vi "Lockin_Amplifier_diag_realtime.vi"(0 "Second":bool, 1 "Sample Number":i32=100000, 2 "all rows":dbl[][](array[numeric]) format="%0.3f", 3 "Cutoff Frequency":dbl=500.0, 4 "dt":dbl=0.0002, 5 "Window (s)":dbl=3.0, 7 "Resolution":dbl=0.0001, 8 "averaging time":dbl=1.0 format="%0.2p", 9 "Error In":errorcluster, 12 "Sampling Freq":dbl=5000.0, 14 "tolerance (Deviation)":dbl=3.0) -> (13 "Error Out":errorcluster, 15 "dLD_RMS":dbl, 16 "LD_RMS":dbl, 17 "Signal Spectrum":cluster{"f0":dbl, "df":dbl, "magnitude":dbl[]}[](graph), 20 "Lock-in R (Vrms)":cluster{dbl[], "Result":dbl[]}(graph), 21 "Lock-in Theta":cluster{dbl[], "Result":dbl[]}(graph), 23 "Time Domain Signal":cluster{"xi used":dbl[], "yi":dbl[]}[](graph), 24 "Phase average":dbl format="%0.2f", 25 "Phase  deviation":dbl format="%0.2f", 27 "Integral":cluster{dbl[], dbl[]}[](graph))   [LabVIEW 2013]
uses:
  <vilib>/gmath/NI_Gmath.lvlib
  <vilib>/Analysis/NI_AALBase.lvlib
panel:
  out "Averaging window":dbl
  in  "Tab Control":T1(tab)
  out "Reference signal / PLL Signal":cluster{"all rows":dbl[], "all rows":dbl[]}[](graph)
  out "Reference Spectrum":cluster{"f0":dbl, "df":dbl, "magnitude":dbl[]}(graph)
  out "Synthetized Spectrum":cluster{"f0":dbl, "df":dbl, "magnitude":dbl[]}(graph)
  in  "t0_ref":dbl
  in  "t0_LD":dbl=0.0001
  out "LD Spectrum":cluster{"f0":dbl, "df":dbl, "magnitude":dbl[]}(graph)
  out "LD Signal":cluster{"all rows":dbl[], "all rows":dbl[]}[](graph)
  out "Tolerance Level":dbl
  out "average":dbl
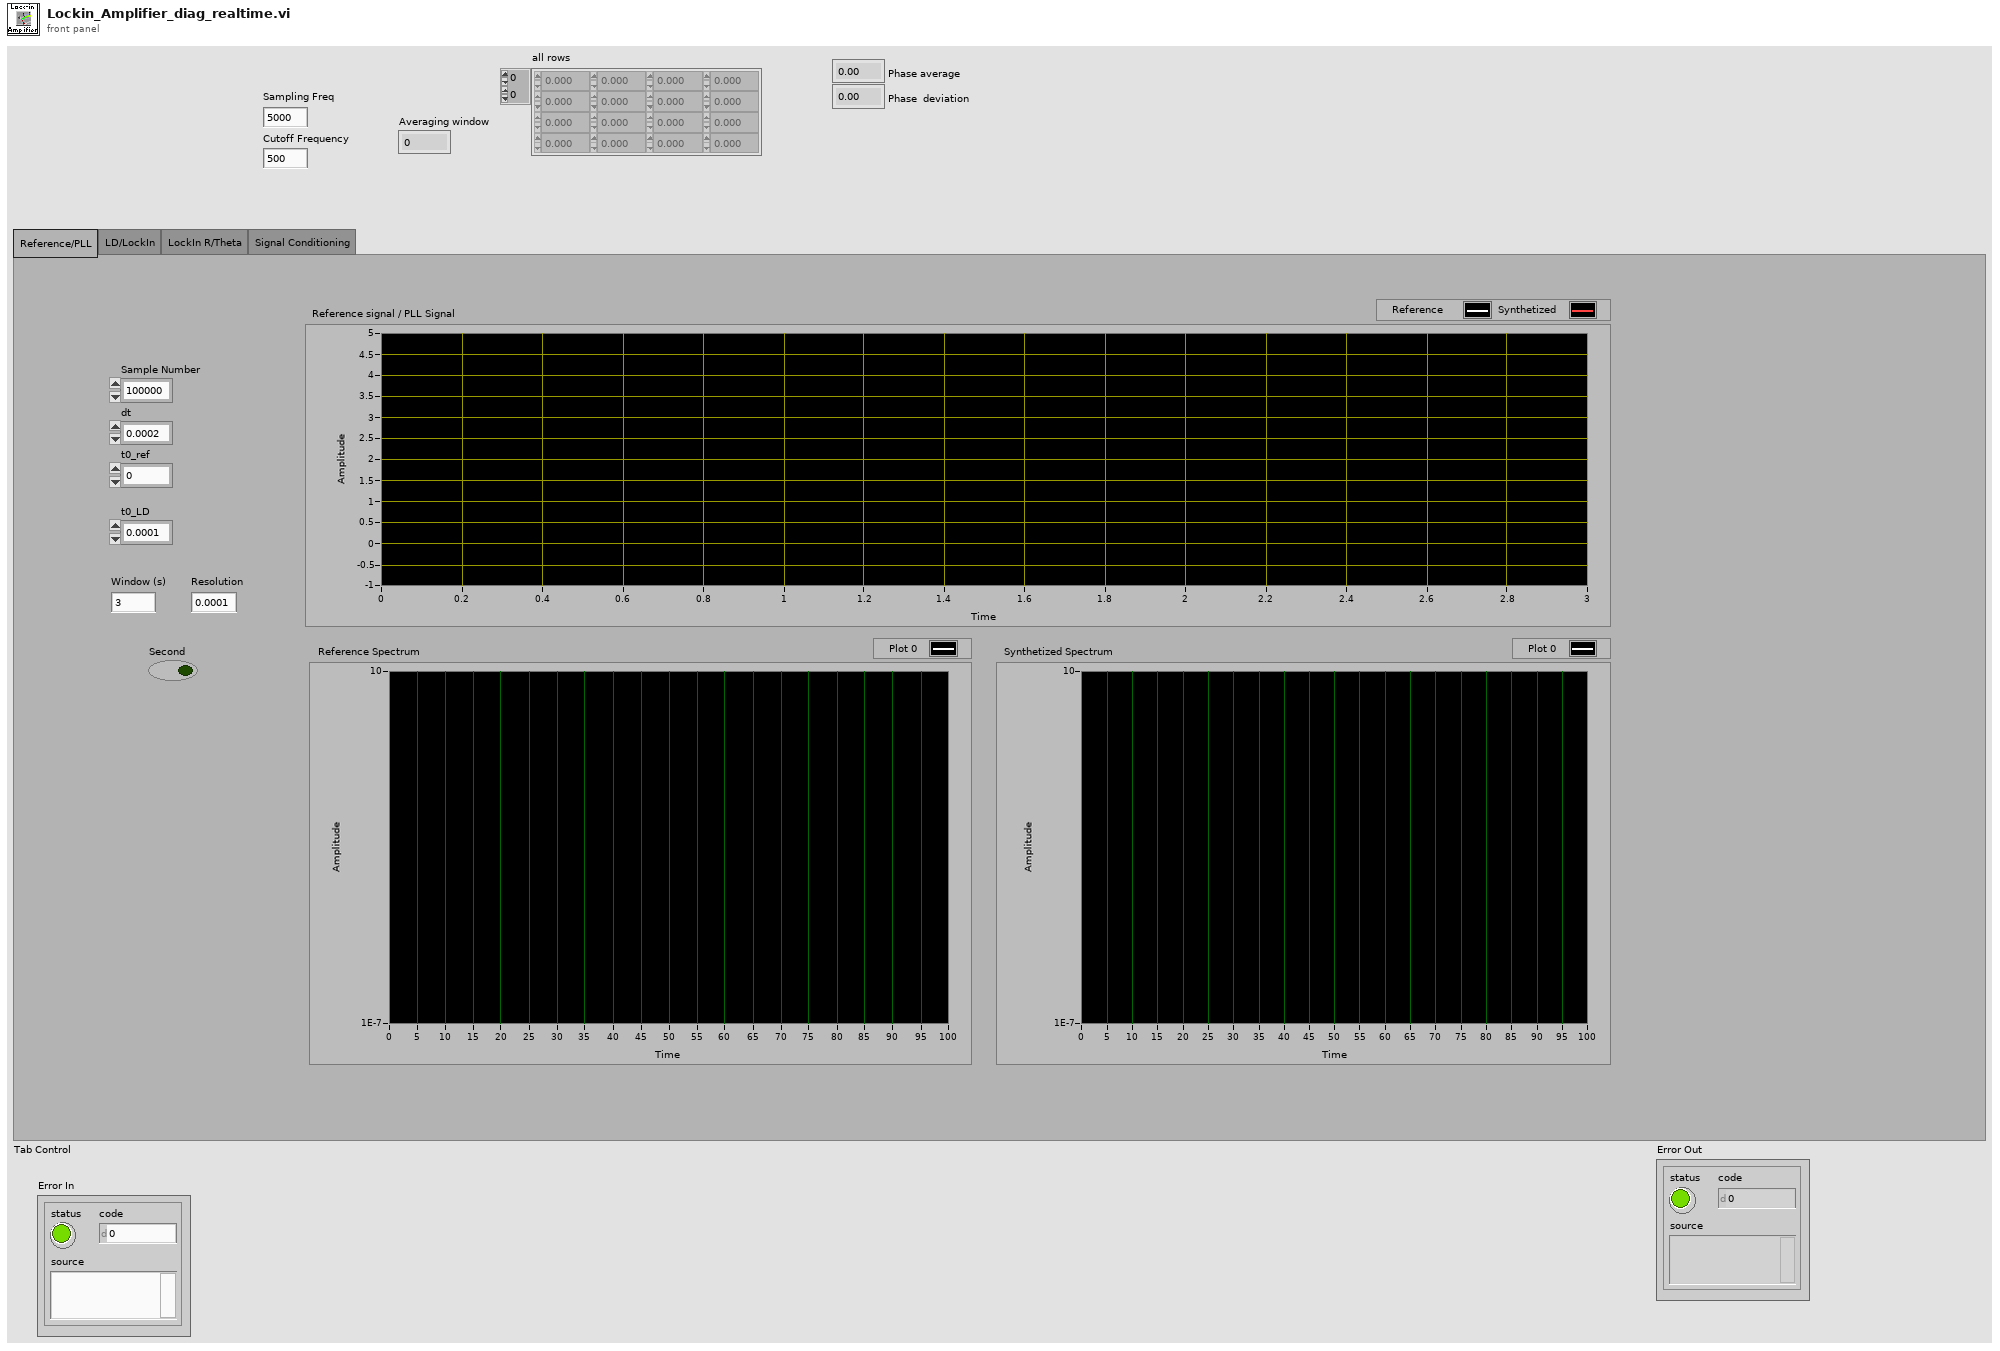
[diagram p1: front panel]
types:
  T1 = enum32{"Reference/PLL", "LD/LockIn", "LockIn R/Theta", "Signal Conditioning"}
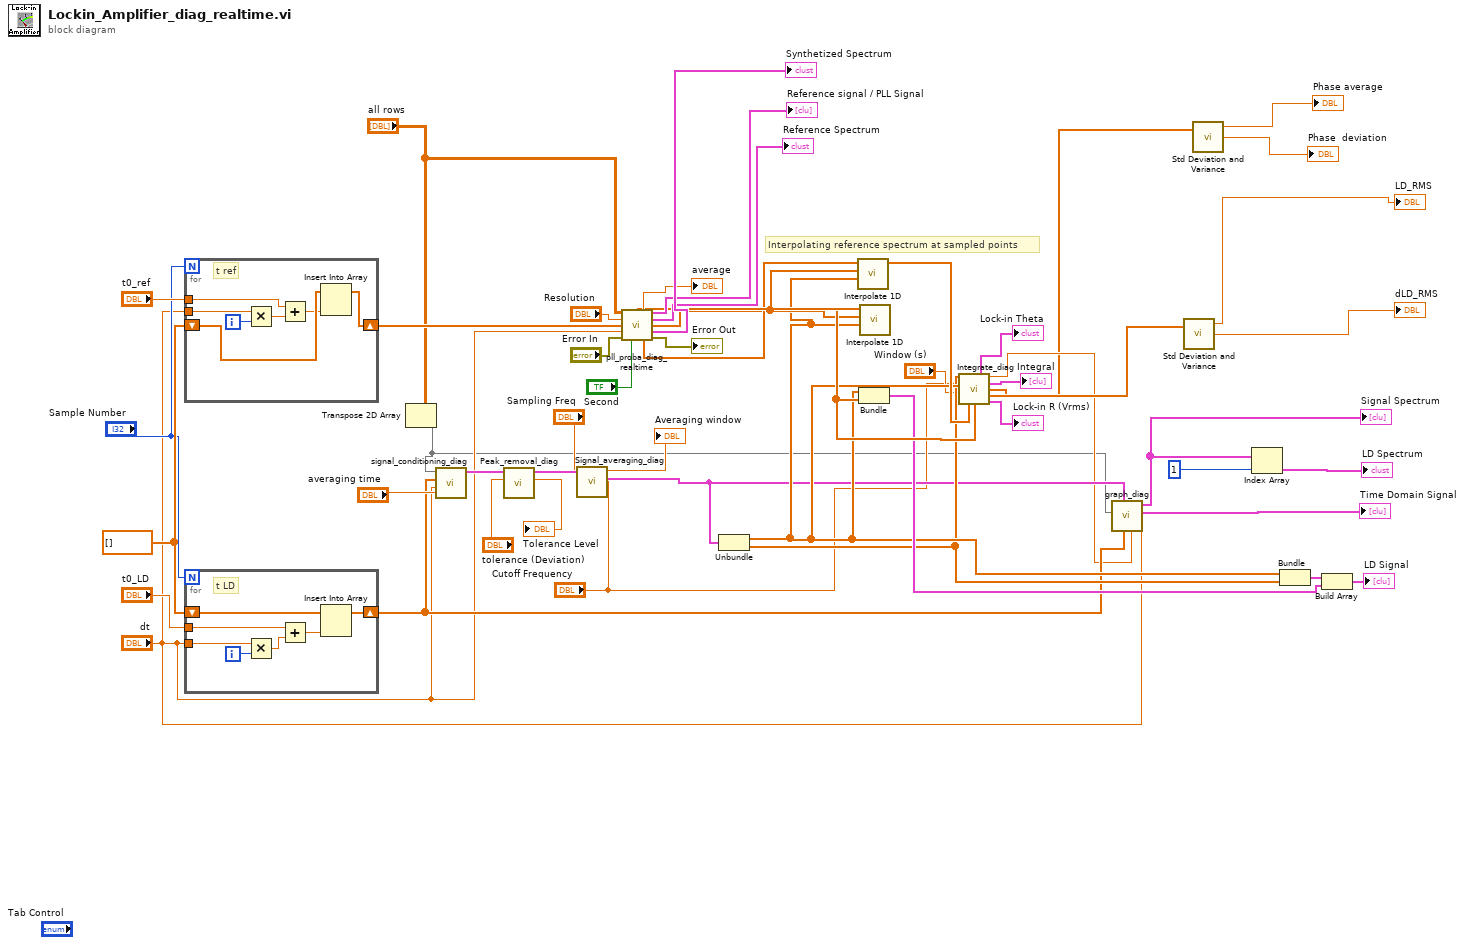
[diagram p0: block diagram]
diagram:
  w26 = dbl[] []
  # "Interpolating reference spectrum at sampled points"
  n1 = for {
    N: "Sample Number" -> [_]
    shift-right: [w57] -> w27
    shift-left: w26 -> [w56]
    tunnel: "dt" -> [w55]
    tunnel: "t0_ref" -> [w54]
    i -> [w58]
    # "t ref"
    n2 = Multiply(x=w55, y=w58) -> (x*y=w53:dbl)
    n3 = Add(x=w54, y=w53) -> (x+y=w52:dbl)
    n4 = Insert Into Array(array=w56, new element=w52) -> (w57:dbl[])  [unwired: 1 in]
  }
  n5 = for {
    N: "Sample Number" -> [_]
    shift-right: [w64] -> w23
    shift-left: w26 -> [w63]
    tunnel: "dt" -> [w62]
    tunnel: "t0_LD" -> [w61]
    i -> [w65]
    # "t LD"
    n6 = Multiply(x=w62, y=w65) -> (x*y=w60:dbl)
    n7 = Add(x=w61, y=w60) -> (x+y=w59:dbl)
    n8 = Insert Into Array(array=w63, new element=w59) -> (w64:dbl[])  [unwired: 1 in]
  }
  n9 = Transpose 2D Array(2D array="all rows") -> (transposed array=w2:dbl[][])
  n10 = call "signal_conditioning_diag.vi"("averaging time"="averaging time", "dt"="dt", "t_LD"=w23, "all rows"=w2) -> ("Offset removed"=w29:cluster{"xi used":dbl[], "yi":dbl[]})  [unwired: 6 in, 1 out]
  n11 = call "Peak_removal_diag.vi"("tolerance (Deviation)"="tolerance (Deviation)", "Offset removed"=w29) -> ("Tolerance Level"=→"Tolerance Level":dbl, "XY Graph"=w20:cluster{"xi used":dbl[], "yi":dbl[]})  [unwired: 8 in]
  n12 = call "Signal_averaging_diag.vi"("Pike removed"=w20, "Cutoff Frequency"="Cutoff Frequency", "Sampling Freq"="Sampling Freq") -> ("Averaged"=w19:cluster{"xi used":dbl[], "yi":dbl[]}, "Averaging window"=→"Averaging window":dbl)  [unwired: 7 in]
  n13 = call "pll_proba_diag_realtime.vi"("all rows"="all rows", "Resolution"="Resolution", "t_ref"=w27, "dt"="dt", "Error In"="Error In", "Second"="Second") -> ("average"=→"average":dbl, "XY Graph"=→"Reference signal / PLL Signal":cluster{"all rows":dbl[], "all rows":dbl[]}[], "Waveform Graph"=→"Reference Spectrum":cluster{"f0":dbl, "df":dbl, "magnitude":dbl[]}, "time"=w37:dbl[], "Waveform Graph 2"=→"Synthetized Spectrum":cluster{"f0":dbl, "df":dbl, "magnitude":dbl[]}, "PLL_sine"=w41:dbl[], "PLL_cosine"=w38:dbl[], "Error Out"=→"Error Out":errorcluster)  [unwired: 2 in]
  n14 = Unbundle(w19) -> ("xi used"=w33:dbl[], "yi"=w32:dbl[])
  n15 = call <vilib>:"Interpolate 1D.vi"("xi"=w33, "X"=w37, "Y"=w38) -> ("yi"=w36:dbl[])  [unwired: 6 in, 2 out]
  n16 = call <vilib>:"Interpolate 1D.vi"("xi"=w33, "X"=w37, "Y"=w41) -> ("yi"=w40:dbl[])  [unwired: 6 in, 2 out]
  n17 = Bundle("xi used"=w33, "yi"=w40) -> (w39:cluster{"xi used":dbl[], "yi":dbl[]})  [unwired: 1 in]
  n18 = call "Integrate_diag.vi"("Processed LD values"=w32, "Processed LD time values"=w33, "Cutoff Frequency"="Cutoff Frequency", "Window (s)"="Window (s)", "Ref Sine"=w36, "Ref Cosine"=w40) -> ("Lockin Theta"=→"Lock-in Theta":cluster{dbl[], "Result":dbl[]}, "Numeric"=w14:dbl, "Lock in X,Y,R (Vrms) time"=→"Integral":cluster{dbl[], "Result":dbl[]}[], "LockIn Theta Array"=w9:dbl[], "LockIn R (Vrms) array"=w21:dbl[], "LockIn R (Vrms)"=→"Lock-in R (Vrms)":cluster{dbl[], "Result":dbl[]})  [unwired: 3 in, 1 out]
  n19 = call "graph_diag.vi"(4:"dt"=w14, "Array in"=w23, "Averaged"=w19, "LD Timetrace in"=w2, 11:"dt"="dt") -> ("Time Domain Signal"=→"Time Domain Signal":cluster{"xi used":dbl[], "yi":dbl[]}[], "Spectra"=w12:cluster{"f0":dbl, "df":dbl, "magnitude":dbl[]}[])  [unwired: 5 in]
  "Signal Spectrum" <- w12
  n20 = call <vilib>:"Std Deviation and Variance.vi"("X"=w21) -> ("mean"=→"LD_RMS":dbl, "standard deviation"=→"dLD_RMS":dbl)  [unwired: 1 in, 1 out]
  n21 = call <vilib>:"Std Deviation and Variance.vi"("X"=w9) -> ("mean"=→"Phase average":dbl, "standard deviation"=→"Phase  deviation":dbl)  [unwired: 1 in, 1 out]
  n22 = Index Array(array=w12, index=1) -> (element=→"LD Spectrum":cluster{"f0":dbl, "df":dbl, "magnitude":dbl[]})
  n23 = Bundle("xi used"=w33, "yi"=w32) -> (w42:cluster{"xi used":dbl[], "yi":dbl[]})  [unwired: 1 in]
  n24 = Build Array(w42, w39) -> (→"LD Signal":cluster{"xi used":dbl[], "yi":dbl[]}[])
